vi "test Clear Data.vi"(8 "error in (no error)":errorcluster, 11 "TestCase in":refnum<class "Data Manipulation Tests.lvclass">) -> (0 "error out":errorcluster, 3 "TestCase out":refnum<class "Data Manipulation Tests.lvclass">)   [LabVIEW 2017, in "Pointer Tests.lvlib" / "Data Manipulation Tests.lvclass"]
uses:
  Data Manipulation Tests.lvclass
  Source/Classes/Pointer/Public/New/New (1B).vi
  Source/Classes/Pointer/Public/Write/Write (1D U8).vi
  Source/Classes/Pointer/Public/Read/Read (1D U8).vi
  <vilib>/addons/_JKI Toolkits/VI Tester/TestCase.llb/TestCase.lvclass
  Source/Classes/Pointer/Pointer.lvclass
  C:/Program Files (x86)/National Instruments/LabVIEW 2017/vi.lib/addons/_JKI Toolkits/VI Tester/TestCase.llb/TestCase.lvclass
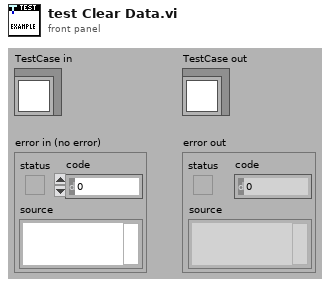
[diagram p1: front panel]
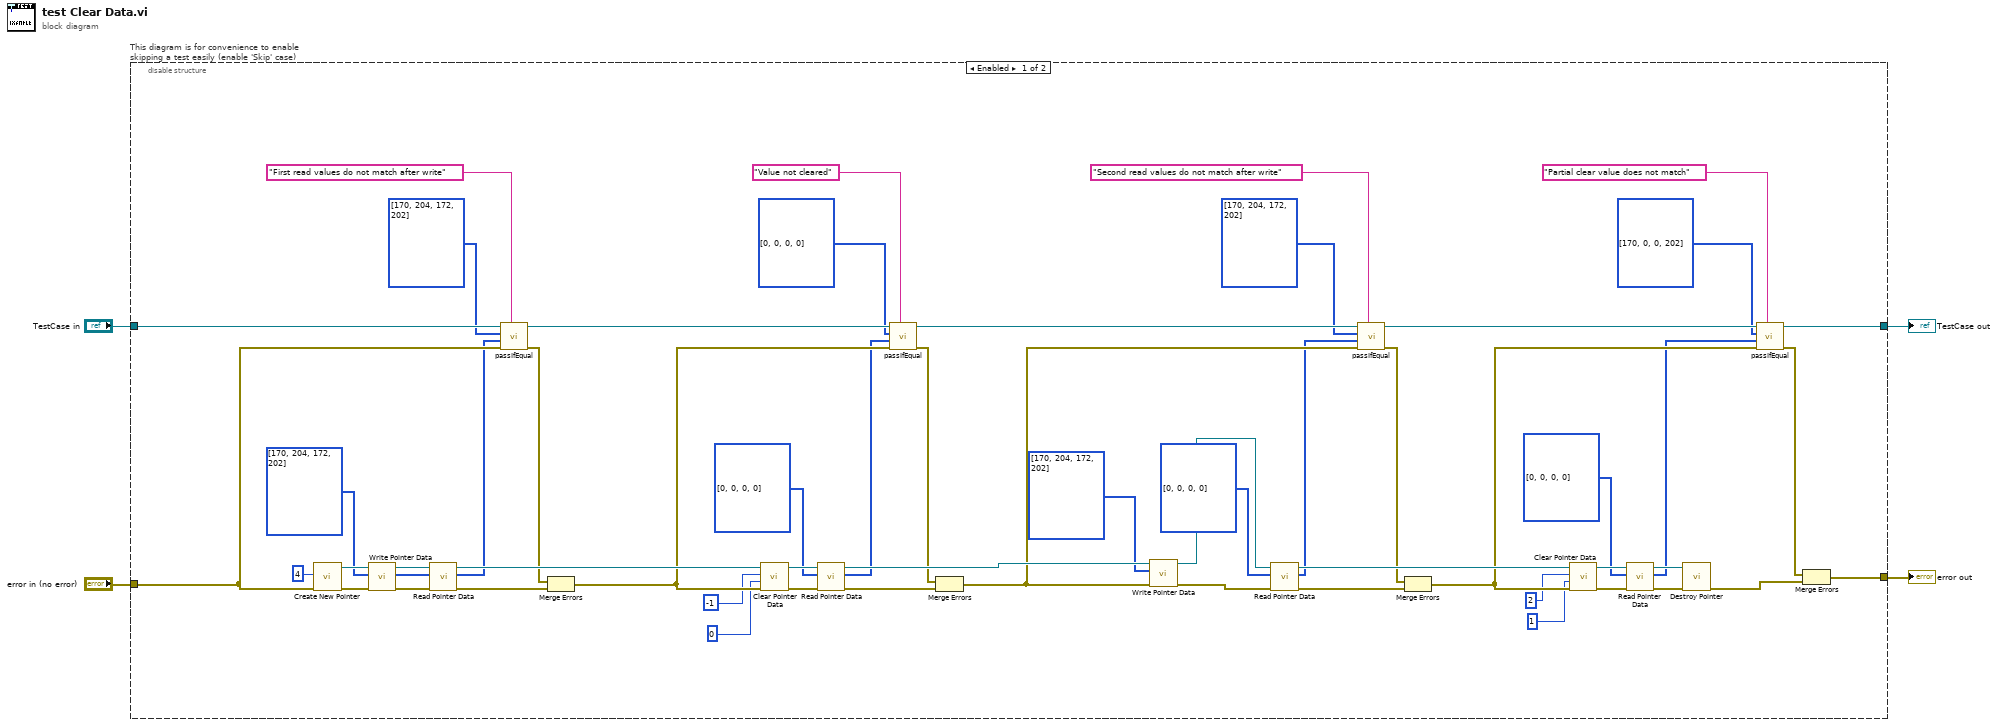
[diagram p0: block diagram]
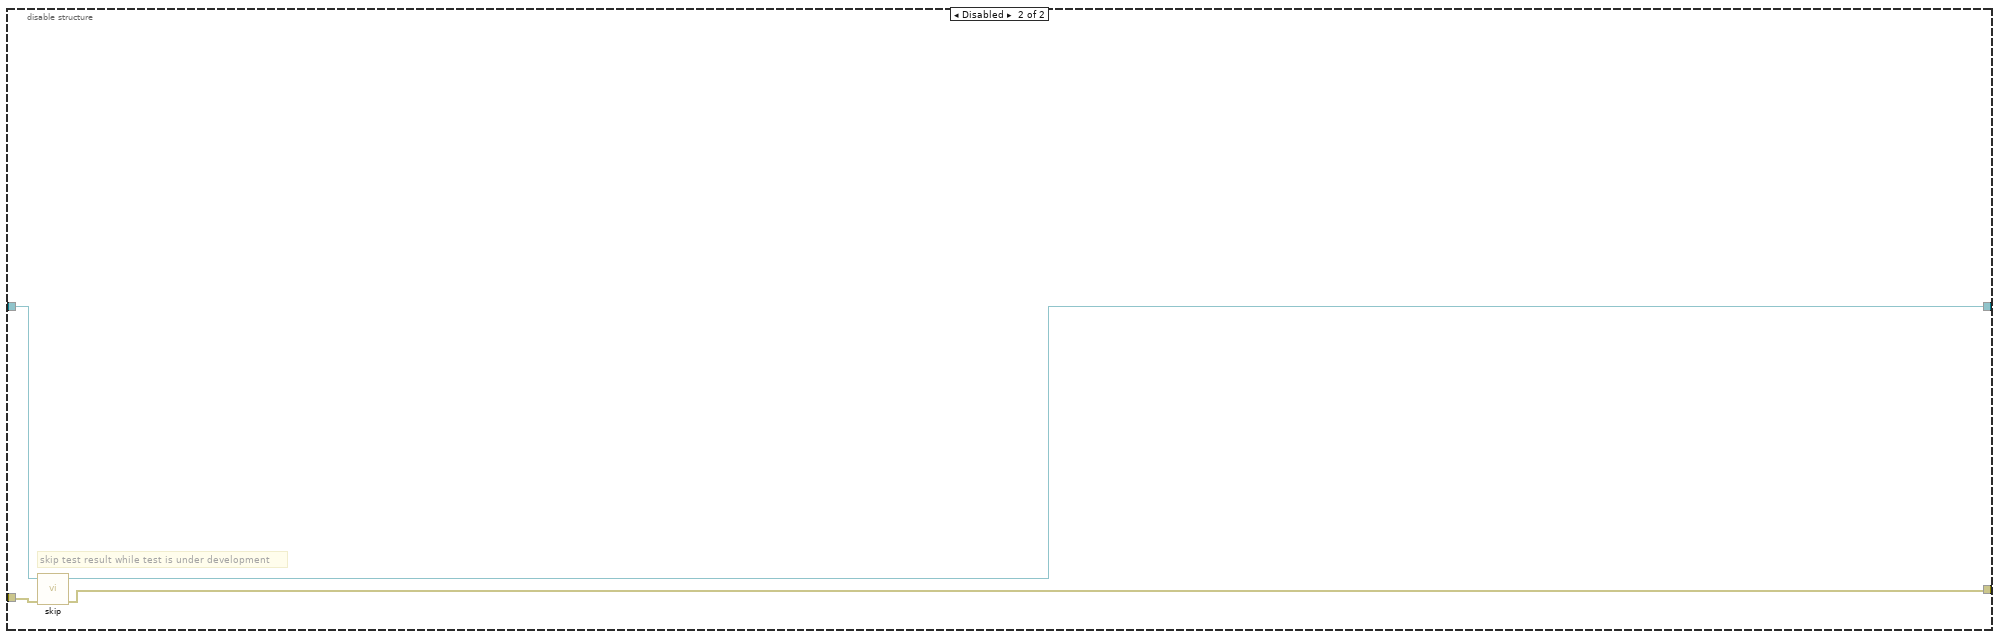
[diagram p2: hidden frame]
diagram:
  n1 = disable-structure "This diagram is for convenience to enable skipping a test easily (enable 'Skip' case)" shown="Enabled" {
    disable-tunnel: "TestCase in" -> [w56 w64]
    disable-tunnel: [w59 w62] -> w1
    disable-tunnel: [w58 w63] -> w3
    disable-tunnel: "error in (no error)" -> [w51 w61]
    frame Enabled {
      n2 = call-poly "Create New Pointer.vi"("error in (no error)"=w51, "count (1)"=u64 4) -> ("error out"=w45:errorcluster, "Pointer"=w47:refnum<class "Pointer.lvclass">)  [unwired: 8 in]
      n3 = call-poly "Write Pointer Data.vi"("error in (no error)"=w45, "buffer in"=u8[] [170, 204, 172, 202], "Pointer in"=w47) -> ("error out"=w44:errorcluster, "buffer out"=w39:u8[], "Pointer out"=w42:refnum<class "Pointer.lvclass">)  [unwired: 5 in, 1 out]
      n4 = call-poly "Read Pointer Data.vi"("error in (no error)"=w44, "buffer in"=w39, "Pointer in"=w42) -> ("error out"=w43:errorcluster, "buffer out"=w5:u8[], "Pointer out"=w57:refnum<class "Pointer.lvclass">)  [unwired: 5 in, 1 out]
      n5 = call-dynamic "passIfEqual.vi"("custom report message (\"\")"="First read values do not match after write" ("custom report message (\"\")"), "error in (no error)"=w51, "y"=w5, "x"=u8[] [170, 204, 172, 202] ("buffer in"), "TestCase in"=w56) -> ("error out"=w38:errorcluster, "TestCase out"=w55:refnum<class "Data Manipulation Tests.lvclass">)  [unwired: 5 in]
      n6 = Merge Errors(w38, w43) -> (w50:errorcluster)
      n7 = call "Clear Pointer Data.vi"("error in (no error)"=w50, "offset (0)"=u64 0, "length (-1: rest)"=i64 -1, "Pointer in"=w57) -> ("error out"=w36:errorcluster, "Pointer out"=w35:refnum<class "Pointer.lvclass">)  [unwired: 6 in]
      n8 = call-poly "Read Pointer Data.vi"("error in (no error)"=w36, "buffer in"=u8[] [0, 0, 0, 0], "Pointer in"=w35) -> ("error out"=w37:errorcluster, "buffer out"=w28:u8[], "Pointer out"=w60:refnum<class "Pointer.lvclass">)  [unwired: 5 in, 1 out]
      n9 = call-dynamic "passIfEqual.vi"("custom report message (\"\")"="Value not cleared" ("custom report message (\"\")"), "error in (no error)"=w50, "y"=w28, "x"=u8[] [0, 0, 0, 0] ("buffer in"), "TestCase in"=w55) -> ("error out"=w31:errorcluster, "TestCase out"=w53:refnum<class "Data Manipulation Tests.lvclass">)  [unwired: 5 in]
      n10 = Merge Errors(w31, w37) -> (w49:errorcluster)
      n11 = call-poly "Write Pointer Data.vi"("error in (no error)"=w49, "buffer in"=u8[] [170, 204, 172, 202], "Pointer in"=w60) -> ("error out"=w27:errorcluster, "Pointer out"=w25:refnum<class "Pointer.lvclass">)  [unwired: 5 in, 2 out]
      n12 = call-poly "Read Pointer Data.vi"("error in (no error)"=w27, "buffer in"=u8[] [0, 0, 0, 0], "Pointer in"=w25) -> ("error out"=w26:errorcluster, "buffer out"=w23:u8[], "Pointer out"=w54:refnum<class "Pointer.lvclass">)  [unwired: 5 in, 1 out]
      n13 = call-dynamic "passIfEqual.vi"("custom report message (\"\")"="Second read values do not match after write" ("custom report message (\"\")"), "error in (no error)"=w49, "y"=w23, "x"=u8[] [170, 204, 172, 202] ("buffer in"), "TestCase in"=w53) -> ("error out"=w22:errorcluster, "TestCase out"=w52:refnum<class "Data Manipulation Tests.lvclass">)  [unwired: 5 in]
      n14 = Merge Errors(w22, w26) -> (w48:errorcluster)
      n15 = call "Clear Pointer Data.vi"("error in (no error)"=w48, "offset (0)"=u64 1, "length (-1: rest)"=i64 2, "Pointer in"=w54) -> ("error out"=w16:errorcluster, "Pointer out"=w15:refnum<class "Pointer.lvclass">)  [unwired: 6 in]
      n16 = call-poly "Read Pointer Data.vi"("error in (no error)"=w16, "buffer in"=u8[] [0, 0, 0, 0], "Pointer in"=w15) -> ("error out"=w17:errorcluster, "buffer out"=w7:u8[], "Pointer out"=w10:refnum<class "Pointer.lvclass">)  [unwired: 5 in, 1 out]
      n17 = call "Destroy Pointer.vi"("error in (no error)"=w17, "Pointer in"=w10) -> ("error out"=w11:errorcluster)  [unwired: 8 in, 1 out]
      n18 = call-dynamic "passIfEqual.vi"("custom report message (\"\")"="Partial clear value does not match" ("custom report message (\"\")"), "error in (no error)"=w48, "y"=w7, "x"=u8[] [170, 0, 0, 202] ("buffer in"), "TestCase in"=w52) -> ("error out"=w18:errorcluster, "TestCase out"=w59:refnum<class "Data Manipulation Tests.lvclass">)  [unwired: 5 in]
      n19 = Merge Errors(w18, w11) -> (w58:errorcluster)
    }
    frame Disabled {
      # "skip test result while test is under development"
      n20 = call <vilib>:"skip.vi"("error in (no error)"=w61, "TestCase in"=w64) -> ("error out"=w63:errorcluster, "TestCase out"=w62:refnum<class "Data Manipulation Tests.lvclass">)  [unwired: 8 in]
    }
  }
  "error out" <- w3
  "TestCase out" <- w1
